vi "Generic 2 Axis DAQmx AO Stage Engine.vi"(0 "Unique Notifier Name":string="Not a Name", 11 "DIO Lines":string[](array[string])) -> ()   [LabVIEW 2020]
uses:
  Stages Controls/Stage Notifier Element.ctl
  Stages Controls/Stage Actions.ctl
  Stages Controls/Stage Status.ctl
  <vilib>/DAQmx/write.llb/DAQmx Write (Analog DBL 1Chan 1Samp).vi
  <vilib>/DAQmx/create/channels.llb/DAQmx Create Channel (AO-Voltage-Basic).vi
  <vilib>/DAQmx/miscellaneous.llb/DAQmx Fill In Error Info.vi
panel:
  in  "Quit":bool
  in  "Home":bool
  in  "Get Position":bool
  in  "Position (µm)":dbl format="%#_4g"
  in  "Step Size (µm)":dbl format="%#_4g"
  in  "Up":bool
  in  "Down":bool
  # "Array Elements must be:\n\n1) AO Channel 1 (e.g. Dev1/ao0)\n2) AO Channel 2\n3) Max voltage\n4) Min voltage\n5) Volts/µm"
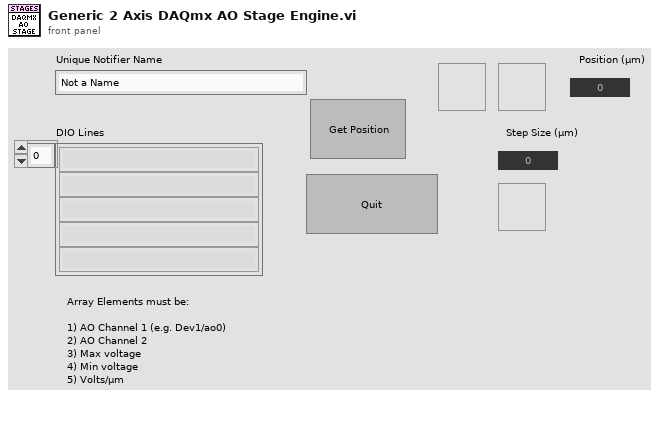
[diagram p1: front panel]
types:
  T1 = typedef "Stage Notifier Element.ctl" = cluster{"Action":T2, "Axis":bool[], "Setpoint":dbl[], "Velocity":dbl, "Cmd Recvd?":bool, "Position":dbl[], "Status":T3, "Misc":variant}
  T2 = typedef "Stage Actions.ctl" = enum16{"Get Position", "MVR", "MOVE", "HALT", "ONTARGET", "ERROR", "REFERENCE", "INIT", "VELOCITY", "STATUS", "EXIT", "HOME", "ZEROPOS", "NANOPOS", "ANALOG", "QUIT"}
  T3 = typedef "Stage Status.ctl" = enum16{"Error", "Abort", "Busy", "On Target"}
  T4 = enum32{"Invalid", "Standard", "Closed", "Hidden", "Minimized", "Maximized"}
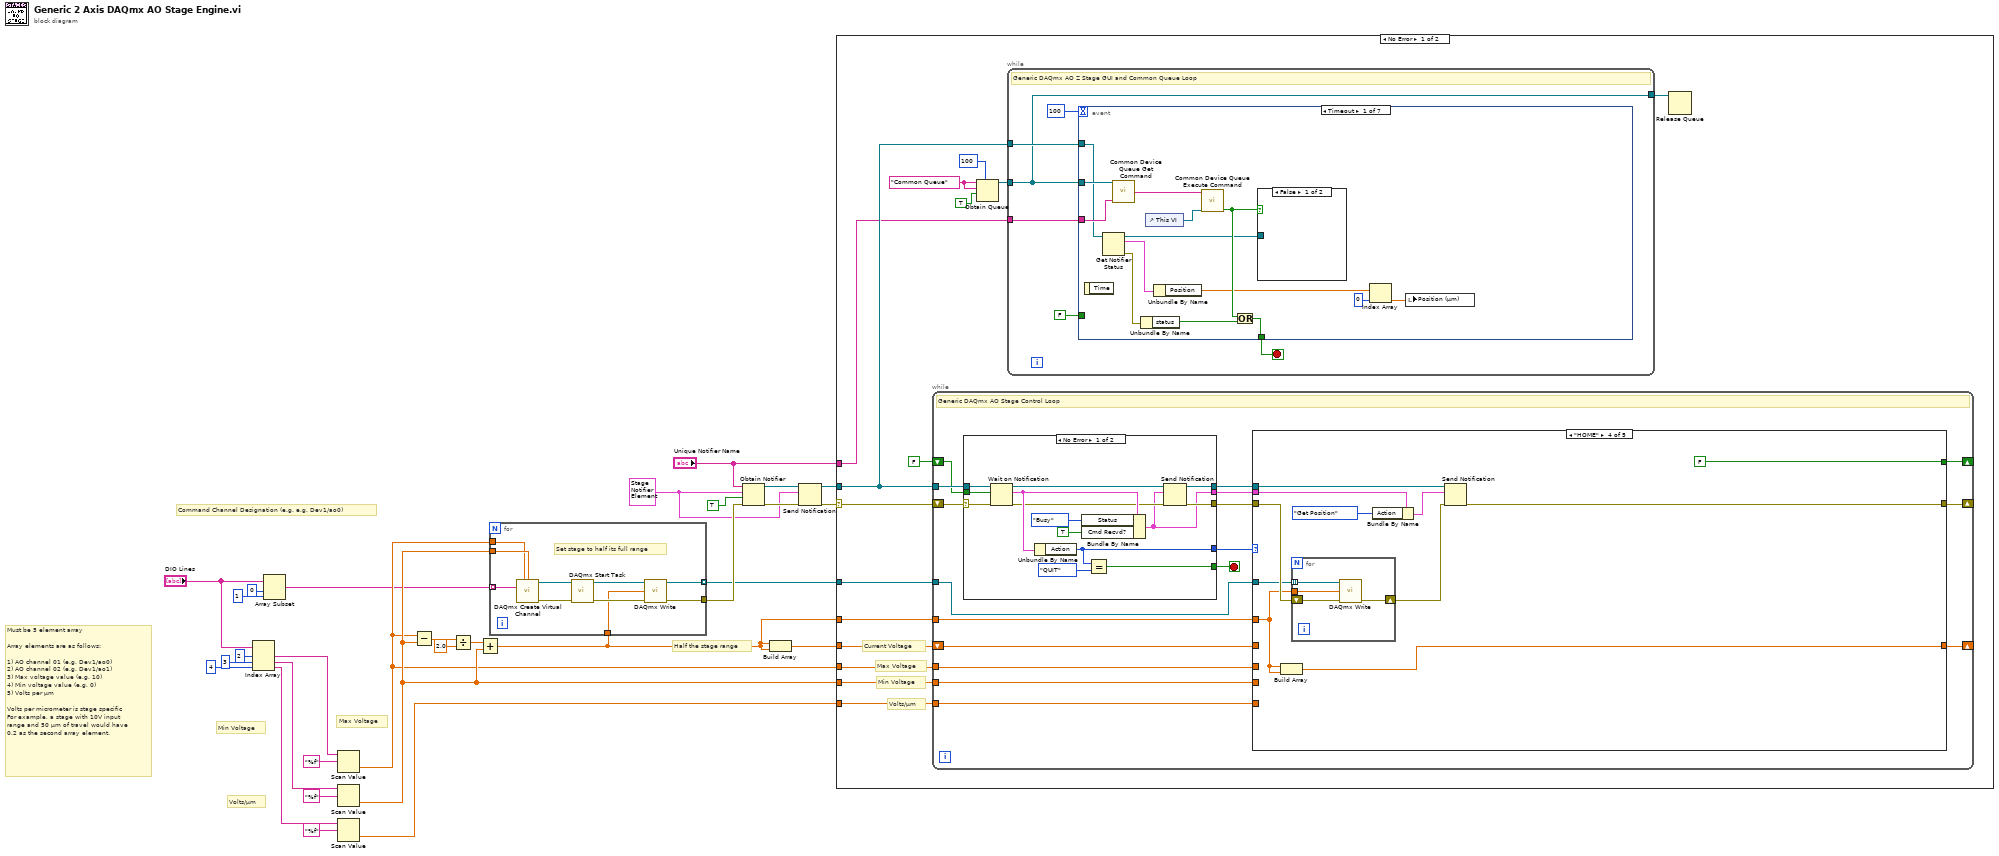
[diagram p0: block diagram]
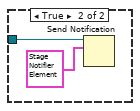
[diagram p2: hidden frame]
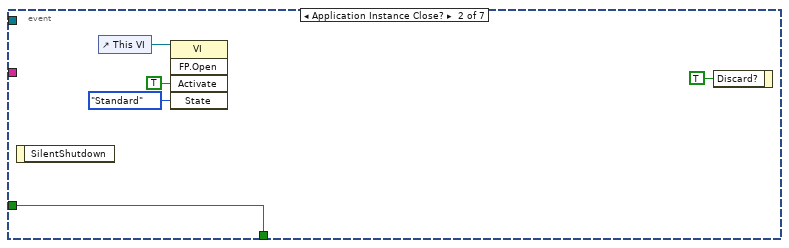
[diagram p3: hidden frame]
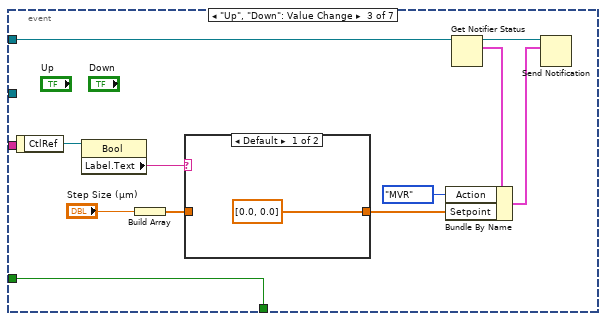
[diagram p4: hidden frame]
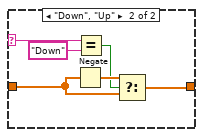
[diagram p5: hidden frame]
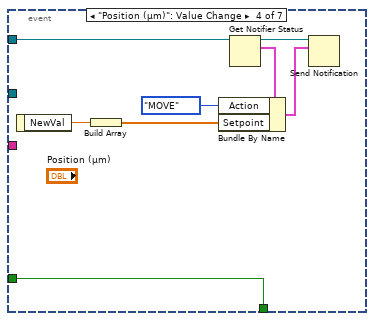
[diagram p6: hidden frame]
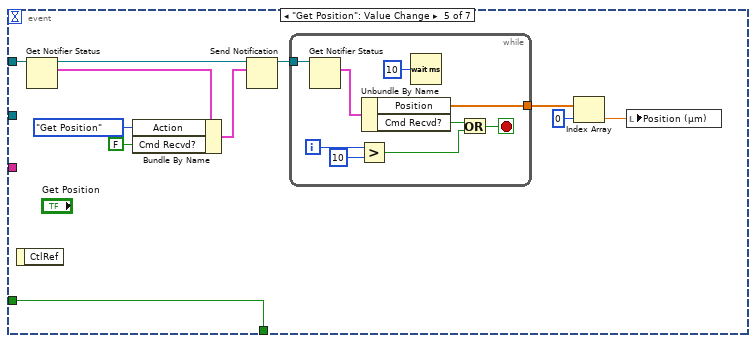
[diagram p7: hidden frame]
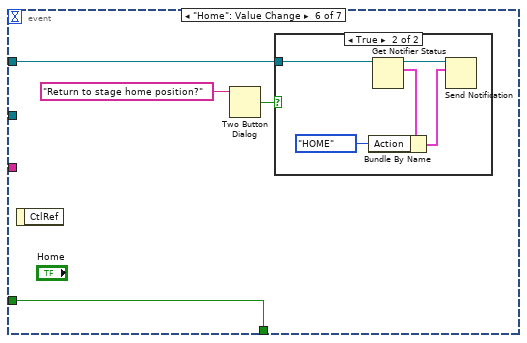
[diagram p8: hidden frame]
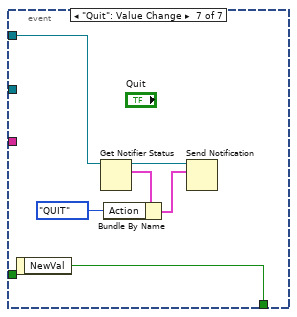
[diagram p10: hidden frame]
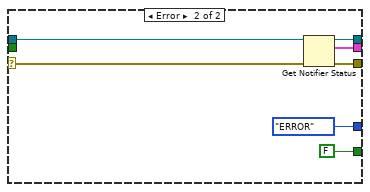
[diagram p11: hidden frame]
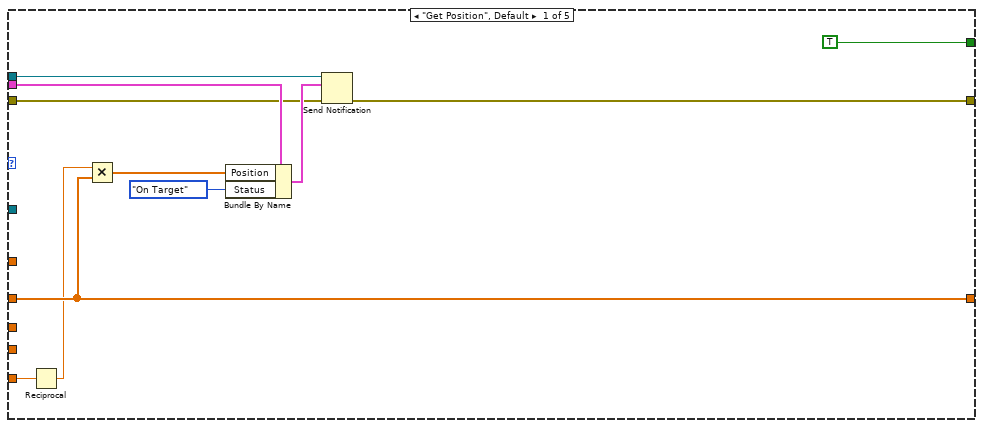
[diagram p12: hidden frame]
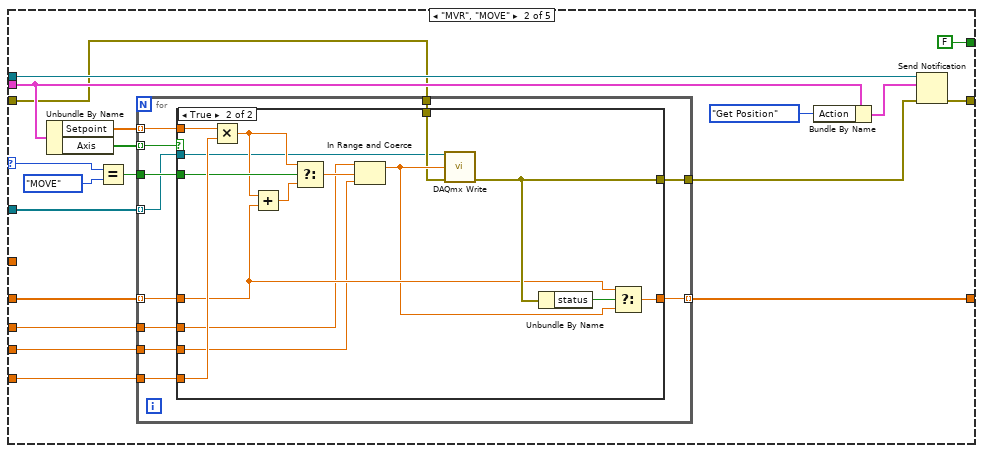
[diagram p13: hidden frame]
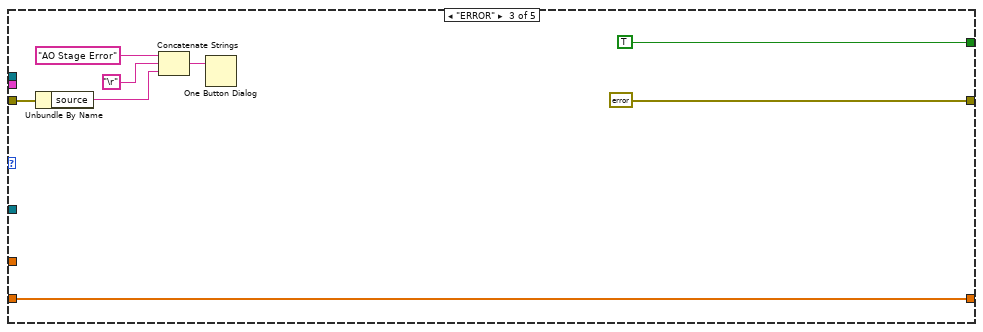
[diagram p15: hidden frame]
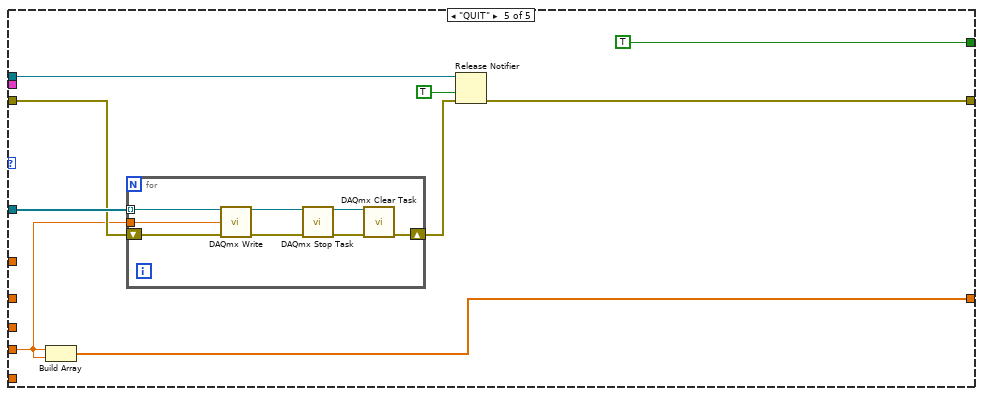
[diagram p16: hidden frame]
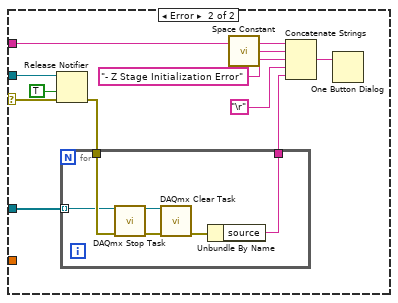
[diagram p17: hidden frame]
diagram:
  w14 = T1 {"Action"=enum."Get Position", "Axis"=[], "Setpoint"=[], "Velocity"=0.5, "Cmd Recvd?"=FALSE, "Position"=[], "Status"=enum."On Target", "Misc"=variant} ("Stage Status")
  # "Half the stage range"
  # "Volts/µm"
  # "Min Voltage"
  # "Max Voltage"
  # "Must be 5 element array\n\nArray elements are as follows:\n\n1) AO channel 01 (e.g. Dev1/ao0)\n2) AO channel 02 (e.g. Dev1/ao1)\n3) Max voltage value (e.g. 10)\n4) Min voltage value (e.g. 0)\n5) Volts per µm\n\nVolts per micrometer is stage specific\nFor example, a stage with 10V input\nrange and 50 µm of travel would have\n0.2 as the second array element."
  # "Command Channel Designation (e.g. e.g. Dev1/ao0)"
  n1 = Index Array(array="DIO Lines", index #1=2 ("index"), index #2=3 ("index"), index #3=4 ("index")) -> (element #1=w6:string, element #2=w5:string, element #3=w4:string)
  n2 = Array Subset(array="DIO Lines", index=0, length=1) -> (w3:string[])
  n3 = Scan Value(string=w6, format string="%f") -> (value=w13:dbl)  [unwired: 1 in, 1 out]
  n4 = Scan Value(string=w5, format string="%f") -> (value=w19:dbl)  [unwired: 1 in, 1 out]
  n5 = Scan Value(string=w4, format string="%f") -> (value=w20:dbl)  [unwired: 1 in, 1 out]
  n6 = Subtract(x=w13, y=w19) -> (x-y=w25:dbl)
  n7 = Divide(x=w25, y=2.0) -> (x/y=w23:dbl)
  n8 = Add(x=w23, y=w19) -> (x+y=w2:dbl)
  n9 = for {
    tunnel: w3 -> [w36] mode=indexing
    tunnel: [w35] -> w26
    tunnel: [w34] -> w21 mode=indexing
    tunnel: w19 -> [w33]
    tunnel: w2 -> [w32]
    tunnel: w13 -> [w31]
    # "Set stage to half its full range"
    n10 = call-poly <vilib>:"DAQmx Create Virtual Channel.vi"("maximum value"=w31, "minimum value"=w33, "physical channels"=w36) -> ("task out"=w39:refnum<k21>, "error out"=w40:errorcluster)  [unwired: 6 in, 5 out]
    n11 = call <vilib>:"DAQmx Start Task.vi"("task/channels in"=w39, "error in"=w40) -> ("task out"=w37:refnum<k21>, "error out"=w38:errorcluster)  [unwired: 12 out]
    n12 = call-poly <vilib>:"DAQmx Write.vi"("task/channels in"=w37, "data"=w32, "error in"=w38) -> ("task out"=w34:refnum<k21>, "error out"=w35:errorcluster)  [unwired: 1 in, 10 out]
  }
  n13 = Obtain Notifier(name (unnamed)="Unique Notifier Name", notification data type=w14, create if not found? (T)=TRUE, error in (no error)=w26) -> (notifier out=w18:refnum<notifier>, error out=w17:errorcluster)  [unwired: 1 out]
  n14 = Build Array(w2, w2) -> (w1:dbl[])
  n15 = Send Notification(notification=w14, notifier=w18, error in (no error)=w17) -> (notifier out=w15:refnum<notifier>, error out=w16:errorcluster)
  n16 = case shown="No Error" w16 {
    selector: w16 -> [w54 w281]
    tunnel: "Unique Notifier Name" -> [w43 w283]
    tunnel: w15 -> [w44 w282]
    tunnel: w21 -> [w55 w280]
    tunnel: w1 -> [w53 _]
    tunnel: w20 -> [w51 _]
    tunnel: w19 -> [w50 _]
    tunnel: w2 -> [w49 _]
    tunnel: w13 -> [w42 _]
    frame No Error {
      w47 = "Common Queue" ("Unique Notifier Name")
      # "Max Voltage"
      # "Current Voltage"
      # "Min Voltage"
      # "Volts/µm"
      n17 = while {
        tunnel: w44 -> [w160]
        tunnel: w55 -> [w146]
        shift-right: [w152] -> _
        shift-left: w53 -> [w153]
        shift-right: [w147] -> _
        shift-left: FALSE -> [w157]
        tunnel: w51 -> [w156]
        tunnel: w50 -> [w155]
        shift-right: [w154] -> _
        shift-left: w54 -> [w145]
        tunnel: w49 -> [w151]
        tunnel: w42 -> [w144]
        stop <- w159 stop-if-true
        # "Generic DAQmx AO Stage Control Loop"
        n18 = case shown="No Error" w145 {
          selector: w145 -> [w161 w179]
          tunnel: w160 -> [w174 w180]
          tunnel: [w172 FALSE] -> w159
          tunnel: [w171 Stage_Actions."ERROR" ("Action")] -> w158
          tunnel: w157 -> [w170 _]
          tunnel: [w166 w178] -> w150
          tunnel: [w165 w176] -> w149
          tunnel: [w163 w177] -> w148
          frame No Error {
            n19 = Wait on Notification(notifier=w174, ignore previous (F)=w170, error in (no error)=w161) -> (notifier out=w167:refnum<notifier>, notification=w169:T1, error out=w164:errorcluster)  [unwired: 1 in, 1 out]
            n20 = Unbundle By Name(w169) -> ("Action"=w171:T2)
            n21 = Bundle By Name(cluster=w169, "Status"=Stage_Status."Busy", "Cmd Recvd?"=TRUE) -> (w163:T1)
            n22 = Equal?(x=w171, y=Stage_Actions."QUIT") -> (x = y?=w172:bool)
            n23 = Send Notification(notification=w163, notifier=w167, error in (no error)=w164) -> (notifier out=w166:refnum<notifier>, error out=w165:errorcluster)
          }
          frame Error {
            n24 = Get Notifier Status(notifier=w180, error in (no error)=w179) -> (notifier out=w178:refnum<notifier>, current notification=w177:T1, error out=w176:errorcluster)  [unwired: 2 out]
          }
        }
        n25 = case shown="\"HOME\"" w158 {
          selector: w158 -> [_ w211 _ _ _]
          tunnel: w156 -> [w186 w209 _ _ _]
          tunnel: w155 -> [_ w198 _ _ w264]
          tunnel: w150 -> [w192 w205 _ w255 w267]
          tunnel: w146 -> [_ w193 _ w250 w271]
          tunnel: w149 -> [w188 w194 w244 w258 w270]
          tunnel: [w187 w203 errorcluster {"status"=FALSE, "code"=0, "source"=""} ("Error") w252 w266] -> w154
          tunnel: w148 -> [w191 w207 _ w257 _]
          tunnel: w153 -> [w185 w200 w247 _ _]
          tunnel: [w185 w199 w247 w248 w263] -> w152
          tunnel: w151 -> [_ _ _ w249 _]
          tunnel: [TRUE FALSE TRUE FALSE TRUE] -> w147
          tunnel: w144 -> [_ w197 _ _ _]
          frame "Get Position", Default {
            n26 = Reciprocal(x=w186) -> (1/x=w184:dbl)
            n27 = Multiply(x=w184, y=w185) -> (x*y=w182:dbl[])
            n28 = Bundle By Name(cluster=w191, "Position"=w182, "Status"=Stage_Status."On Target") -> (w190:T1)
            n29 = Send Notification(notification=w190, notifier=w192, error in (no error)=w188) -> (error out=w187:errorcluster)  [unwired: 1 out]
          }
          frame "MVR", "MOVE" {
            n30 = Unbundle By Name(w207) -> ("Setpoint"=w196:dbl[], "Axis"=w195:bool[])
            n31 = Equal?(x=w211, y=Stage_Actions."MOVE") -> (x = y?=w208:bool)
            n32 = for {
              tunnel: w209 -> [w222]
              tunnel: w208 -> [w221]
              tunnel: [w220] -> w201
              tunnel: w200 -> [w219] mode=indexing
              tunnel: [w218] -> w199 mode=indexing
              tunnel: w198 -> [w217]
              tunnel: w197 -> [w216]
              tunnel: w196 -> [w215] mode=indexing
              tunnel: w195 -> [w214] mode=indexing
              tunnel: w194 -> [w213]
              tunnel: w193 -> [w212] mode=indexing
              n33 = case shown="True" w214 {
                tunnel: w222 -> [_ w239]
                tunnel: w221 -> [_ w238]
                tunnel: [w223 w235] -> w220
                tunnel: w219 -> [w224 w233]
                tunnel: [w224 w232] -> w218
                tunnel: w217 -> [_ w229]
                tunnel: w216 -> [_ w228]
                tunnel: w215 -> [_ w227]
                tunnel: w213 -> [w223 w226]
                tunnel: w212 -> [_ w225]
                frame False {
                }
                frame True {
                  n34 = Multiply(x=w227, y=w239) -> (x*y=w236:dbl)
                  n35 = Add(x=w236, y=w233) -> (x+y=w237:dbl)
                  n36 = Select(t=w236, s=w238, f=w237) -> (s? t:f=w231:dbl)
                  n37 = In Range and Coerce(upper limit=w228, x=w231, lower limit=w229) -> (coerced(x)=w230:dbl)  [unwired: 1 out]
                  n38 = call-poly <vilib>:"DAQmx Write.vi"("task/channels in"=w225, "data"=w230, "error in"=w226) -> ("error out"=w235:errorcluster)  [unwired: 1 in, 11 out]
                  n39 = Unbundle By Name(w235) -> ("status"=w234:bool)
                  n40 = Select(t=w233, s=w234, f=w230) -> (s? t:f=w232:dbl)
                }
              }
            }
            n41 = Bundle By Name(cluster=w207, "Action"=Stage_Actions."Get Position") -> (w204:T1)
            n42 = Send Notification(notification=w204, notifier=w205, error in (no error)=w201) -> (error out=w203:errorcluster)  [unwired: 1 out]
          }
          frame "ERROR" {
            n43 = Unbundle By Name(w244) -> ("source"=w241:string)
            n44 = Concatenate Strings("AO Stage Error" ("message"), "\r", w241) -> (w240:string)
            n45 = One Button Dialog(message=w240) -> ()  [unwired: 1 in, 1 out]
          }
          frame "HOME" {
            n46 = Build Array(w249, w249) -> (w248:dbl[])
            n47 = for {
              tunnel: w250 -> [w260] mode=indexing
              tunnel: w249 -> [w259]
              shift-right: [w261] -> w254
              shift-left: w258 -> [w262]
              n48 = call-poly <vilib>:"DAQmx Write.vi"("task/channels in"=w260, "data"=w259, "error in"=w262) -> ("error out"=w261:errorcluster)  [unwired: 1 in, 11 out]
            }
            n49 = Bundle By Name(cluster=w257, "Action"=Stage_Actions."Get Position") -> (w253:T1)
            n50 = Send Notification(notification=w253, notifier=w255, error in (no error)=w254) -> (error out=w252:errorcluster)  [unwired: 1 out]
          }
          frame "QUIT" {
            n51 = Build Array(w264, w264) -> (w263:dbl[])
            n52 = for {
              tunnel: w271 -> [w279] mode=indexing
              tunnel: w264 -> [w278]
              shift-right: [w272] -> w268
              shift-left: w270 -> [w273]
              n53 = call-poly <vilib>:"DAQmx Write.vi"("task/channels in"=w279, "data"=w278, "error in"=w273) -> ("task out"=w277:refnum<k21>, "error out"=w275:errorcluster)  [unwired: 1 in, 10 out]
              n54 = call <vilib>:"DAQmx Stop Task.vi"("task/channels in"=w277, "error in"=w275) -> ("task out"=w276:refnum<k21>, "error out"=w274:errorcluster)  [unwired: 12 in]
              n55 = call <vilib>:"DAQmx Clear Task.vi"("task in"=w276, "error in"=w274) -> ("error out"=w272:errorcluster)  [unwired: 13 in]
            }
            n56 = Release Notifier(notifier=w267, force destroy? (F)=TRUE, error in (no error)=w268) -> (error out=w266:errorcluster)  [unwired: 2 out]
          }
        }
      }
      n57 = Obtain Queue(max queue size (-1, unlimited)=100, name (unnamed)=w47, element data type=w47, create if not found? (T)=TRUE) -> (queue out=w48:refnum<queue>)  [unwired: 1 in, 2 out]
      n58 = while {
        tunnel: w48 -> [w56]
        tunnel: w43 -> [w59]
        tunnel: w44 -> [w60]
        tunnel: [w56] -> w41
        stop <- w58 stop-if-true
        # "Generic DAQmx AO Z Stage GUI and Common Queue Loop"
        n59 = event shown="[0] Timeout" {
          selector: _ -> [_ _ _ _ _ _ _]
          dyn-events: _ -> [_ _ _ _ _ _ _]
          timeout: 100 -> [_ _ _ _ _ _ _]
          tunnel: w56 -> [w69 _ _ _ _ _ _]
          tunnel: w60 -> [w66 _ w88 w106 w118 w129 w143]
          tunnel: w59 -> [w68 _ _ _ _ _ _]
          tunnel: [w67 w82 w91 w108 w119 w131 w139] -> w58
          tunnel: FALSE -> [_ w82 w91 w108 w119 w131 _]
          event Timeout {
            n60 = event-data() -> ()  [unwired: 1 in, 1 out]
            n61 = Get Notifier Status(notifier=w66) -> (notifier out=w70:refnum<notifier>, current notification=w65:T1, error out=w75:errorcluster)  [unwired: 1 in, 2 out]
            n62 = call "Common Device Queue Get Command.vi"("Common Queue"=w69, "Notifier Name"=w68) -> ("Command"=w74:string)  [unwired: 12 in, 1 out]
            n63 = Unbundle By Name(w75) -> ("status"=w72:bool)
            n64 = control-ref of="This VI"() -> (w73:refnum<vi>)
            n65 = Unbundle By Name(w65) -> ("Position"=w62:dbl[])
            n66 = call "Common Device Queue Execute Command.vi"("Common Command"=w74, "VI Refnum"=w73) -> ("Quit?"=w71:bool)  [unwired: 12 in, 1 out]
            n67 = Or(x=w71, y=w72) -> (x .or. y?=w67:bool)
            n68 = case shown="False" w71 {
              tunnel: w70 -> [_ w77]
              frame False {
              }
              frame True {
                n69 = Send Notification(notification=T1 {"Action"=enum."QUIT", "Axis"=[], "Setpoint"=[], "Velocity"=0.5, "Cmd Recvd?"=FALSE, "Position"=[], "Status"=enum."Error", "Misc"=variant} ("Stage Status"), notifier=w77) -> ()  [unwired: 1 in, 2 out]
              }
            }
            n70 = Index Array(array=w62, index=0) -> (element=w64:dbl)
            n71 = local write "Position (µm)"(w64) -> ()
          }
          event Application Instance Close? {
            n72 = event-data() -> ()  [unwired: 1 in, 1 out]
            n73 = control-ref of="This VI"() -> (w79:refnum<vi>)
            n74 = invoke class="VI" method="FP.Open"(reference=w79, "Activate"=TRUE ("Activate?"), "State"=T4."Standard") -> ()  [unwired: 2 in, 5 out]
            n75 = event-data("Discard?"=TRUE) -> ()  [unwired: 1 in, 1 out]
          }
          event "Up", "Down": Value Change {
            n76 = event-data() -> ("CtlRef"=w90:refnum<vi>)  [unwired: 1 in]
            n77 = property class="Bool"(reference=w90) -> ("Label.Text"=w93:string)  [unwired: 1 in, 2 out]
            n78 = Build Array("Step Size (µm)") -> (w92:dbl[])
            n79 = case shown="Default" w93 {
              selector: w93 -> [_ w100]
              tunnel: w92 -> [_ w97]
              tunnel: [dbl[] [0.0, 0.0] w96] -> w86
              frame Default {
              }
              frame "Down", "Up" {
                n80 = Negate(x=w97) -> (-x=w98:dbl[])
                n81 = Equal?(x=w100, y="Down") -> (x = y?=w95:bool)
                n82 = Select(t=w98, s=w95, f=w97) -> (s? t:f=w96:dbl[])
              }
            }
            n83 = Get Notifier Status(notifier=w88) -> (notifier out=w84:refnum<notifier>, current notification=w87:T1)  [unwired: 1 in, 3 out]
            n84 = Bundle By Name(cluster=w87, "Action"=Stage_Actions."MVR", "Setpoint"=w86) -> (w83:T1)
            n85 = Send Notification(notification=w83, notifier=w84) -> ()  [unwired: 1 in, 2 out]
          }
          event "Position (µm)": Value Change {
            n86 = event-data() -> ("NewVal"=w107:dbl)  [unwired: 1 in]
            n87 = Build Array(w107) -> (w103:dbl[])
            n88 = Get Notifier Status(notifier=w106) -> (notifier out=w105:refnum<notifier>, current notification=w104:T1)  [unwired: 1 in, 3 out]
            n89 = Bundle By Name(cluster=w104, "Action"=Stage_Actions."MOVE", "Setpoint"=w103) -> (w101:T1)
            n90 = Send Notification(notification=w101, notifier=w105) -> ()  [unwired: 1 in, 2 out]
          }
          event "Get Position": Value Change {
            n91 = event-data() -> ()  [unwired: 1 in, 1 out]
            n92 = Get Notifier Status(notifier=w118) -> (notifier out=w117:refnum<notifier>, current notification=w116:T1)  [unwired: 1 in, 3 out]
            n93 = Bundle By Name(cluster=w116, "Action"=Stage_Actions."Get Position", "Cmd Recvd?"=FALSE) -> (w113:T1)
            n94 = Send Notification(notification=w113, notifier=w117) -> (notifier out=w112:refnum<notifier>)  [unwired: 1 in, 1 out]
            n95 = while {
              tunnel: w112 -> [w128]
              tunnel: [w120] -> w111
              i -> [w124]
              stop <- w121 stop-if-true
              n96 = Get Notifier Status(notifier=w128) -> (current notification=w127:T1)  [unwired: 1 in, 4 out]
              n97 = Greater?(x=w124, y=10) -> (0:w122:bool)
              n98 = Unbundle By Name(w127) -> ("Position"=w120:dbl[], "Cmd Recvd?"=w123:bool)
              n99 = Wait (ms)(milliseconds to wait=u32 10) -> ()  [unwired: 1 out]
              n100 = Or(x=w123, y=w122) -> (x .or. y?=w121:bool)
            }
            n101 = Index Array(array=w111, index=0) -> (element=w109:dbl)
            n102 = local write "Position (µm)"(w109) -> ()
          }
          event "Home": Value Change {
            n103 = event-data() -> ()  [unwired: 1 in, 1 out]
            n104 = Two Button Dialog(message="Return to stage home position?") -> (T button?=w130:bool)  [unwired: 2 in]
            n105 = case shown="True" w130 {
              tunnel: w129 -> [_ w137]
              frame False {
              }
              frame True {
                n106 = Get Notifier Status(notifier=w137) -> (notifier out=w136:refnum<notifier>, current notification=w135:T1)  [unwired: 1 in, 3 out]
                n107 = Bundle By Name(cluster=w135, "Action"=Stage_Actions."HOME") -> (w134:T1)
                n108 = Send Notification(notification=w134, notifier=w136) -> ()  [unwired: 1 in, 2 out]
              }
            }
          }
          event "Quit": Value Change {
            n109 = event-data() -> ("NewVal"=w139:bool)  [unwired: 1 in]
            n110 = Get Notifier Status(notifier=w143) -> (notifier out=w142:refnum<notifier>, current notification=w141:T1)  [unwired: 1 in, 3 out]
            n111 = Bundle By Name(cluster=w141, "Action"=Stage_Actions."QUIT") -> (w140:T1)
            n112 = Send Notification(notification=w140, notifier=w142) -> ()  [unwired: 1 in, 2 out]
          }
        }
      }
      n113 = Release Queue(queue=w41) -> ()  [unwired: 2 in, 3 out]
    }
    frame Error {
      n114 = Release Notifier(notifier=w282, force destroy? (F)=TRUE, error in (no error)=w281) -> (error out=w289:errorcluster)  [unwired: 2 out]
      n115 = for {
        tunnel: w289 -> [w294]
        tunnel: [w292] -> w284
        tunnel: w280 -> [w291] mode=indexing
        n116 = call <vilib>:"DAQmx Stop Task.vi"("task/channels in"=w291, "error in"=w294) -> ("task out"=w296:refnum<k21>, "error out"=w295:errorcluster)  [unwired: 12 in]
        n117 = call <vilib>:"DAQmx Clear Task.vi"("task in"=w296, "error in"=w295) -> ("error out"=w293:errorcluster)  [unwired: 13 out]
        n118 = Unbundle By Name(w293) -> ("source"=w292:string)
      }
      n119 = call <vilib>:"Space Constant.vi"() -> ("String"=w287:string)
      n120 = Concatenate Strings(w283, w287, "- Z Stage Initialization Error" ("string"), "\r", w284) -> (w288:string)
      n121 = One Button Dialog(message=w288) -> ()  [unwired: 1 in, 1 out]
    }
  }
